vi "Spiral Search Tool.vi"(7 "Calling VI Ref":refnum<vi>) -> ()   [LabVIEW 2016]
uses:
  Hardware Configuration/Hardware Configuration Controls/Device Type.ctl
  Hardware Configuration/Hardware Configuration Controls/Device Function.ctl
  <vilib>/Utility/miscctls.llb/LVPointTypeDef.ctl
  Spiral Search Tool Type Defs/Spiral Search Tool Notifier Type.ctl
  Spiral Search Tool Type Defs/Spiral Search Tool Actions.ctl
  Device Library/Stages/Stages Controls/Stage Actions.ctl
panel:
  in  "Frames per Step":u32=1
  in  "Step Size (µm)":dbl=1.0
  in  "Camera":i32(ring) items=["Hamamatsu-Camera-Primary-0"]
  in  "Update Cameras":bool
  in  "Exit":bool
  in  "Resume Current":bool
  in  "Pause Current":bool
  in  "Start New":bool
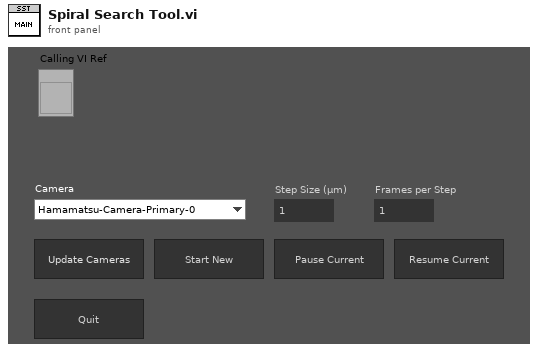
[diagram p1: front panel]
types:
  T1 = enum16{"Always On", "Always Off", "Off While Running"}
  T2 = typedef "LVPointTypeDef.ctl" = cluster{"Horizontal":i16, "Vertical":i16}
  T3 = typedef "Device Function.ctl" = enum16{"Primary", "Secondary", "Overview", "Wide Field Drift Correction", "642 nm Excitation", "560 nm Excitation", "546 nm Excitation", "488 nm Excitation", "405 nm Excitation", "Objective Drift Correction", "Objective XY", "Objective Z", "Sample XY", "Sample Coarse Z", "Sample Z", "4Pi Lower", "4Pi Upper", "Adj Cavity"}
  T4 = typedef "Device Type.ctl" = enum16{"AOTF", "Camera", "Deformable Mirror", "Laser", "Shutter", "Stage"}
  T5 = typedef "Spiral Search Tool Notifier Type.ctl" = cluster{"Actions":T6, "Camera Notifier Name":string}
  T6 = typedef "Spiral Search Tool Actions.ctl" = enum16{"Idle", "Start New", "Resume Current", "Pause Current", "Capture Image", "Move Stage", "Generate Points", "Exit"}
  T7 = typedef "Stage Actions.ctl" = enum16{"Get Position", "MVR", "MOVE", "HALT", "ONTARGET", "ERROR", "REFERENCE", "INIT", "VELOCITY", "STATUS", "EXIT", "HOME", "ZEROPOS", "NANOPOS", "ANALOG", "QUIT"}
  T8 = typedef "LVRectTypeDef.ctl" = cluster{"Left":i16, "Top":i16, "Right":i16, "Bottom":i16}
  T9 = typedef "LVBoundsTypeDef.ctl" = cluster{"Width":u32, "Height":u32}
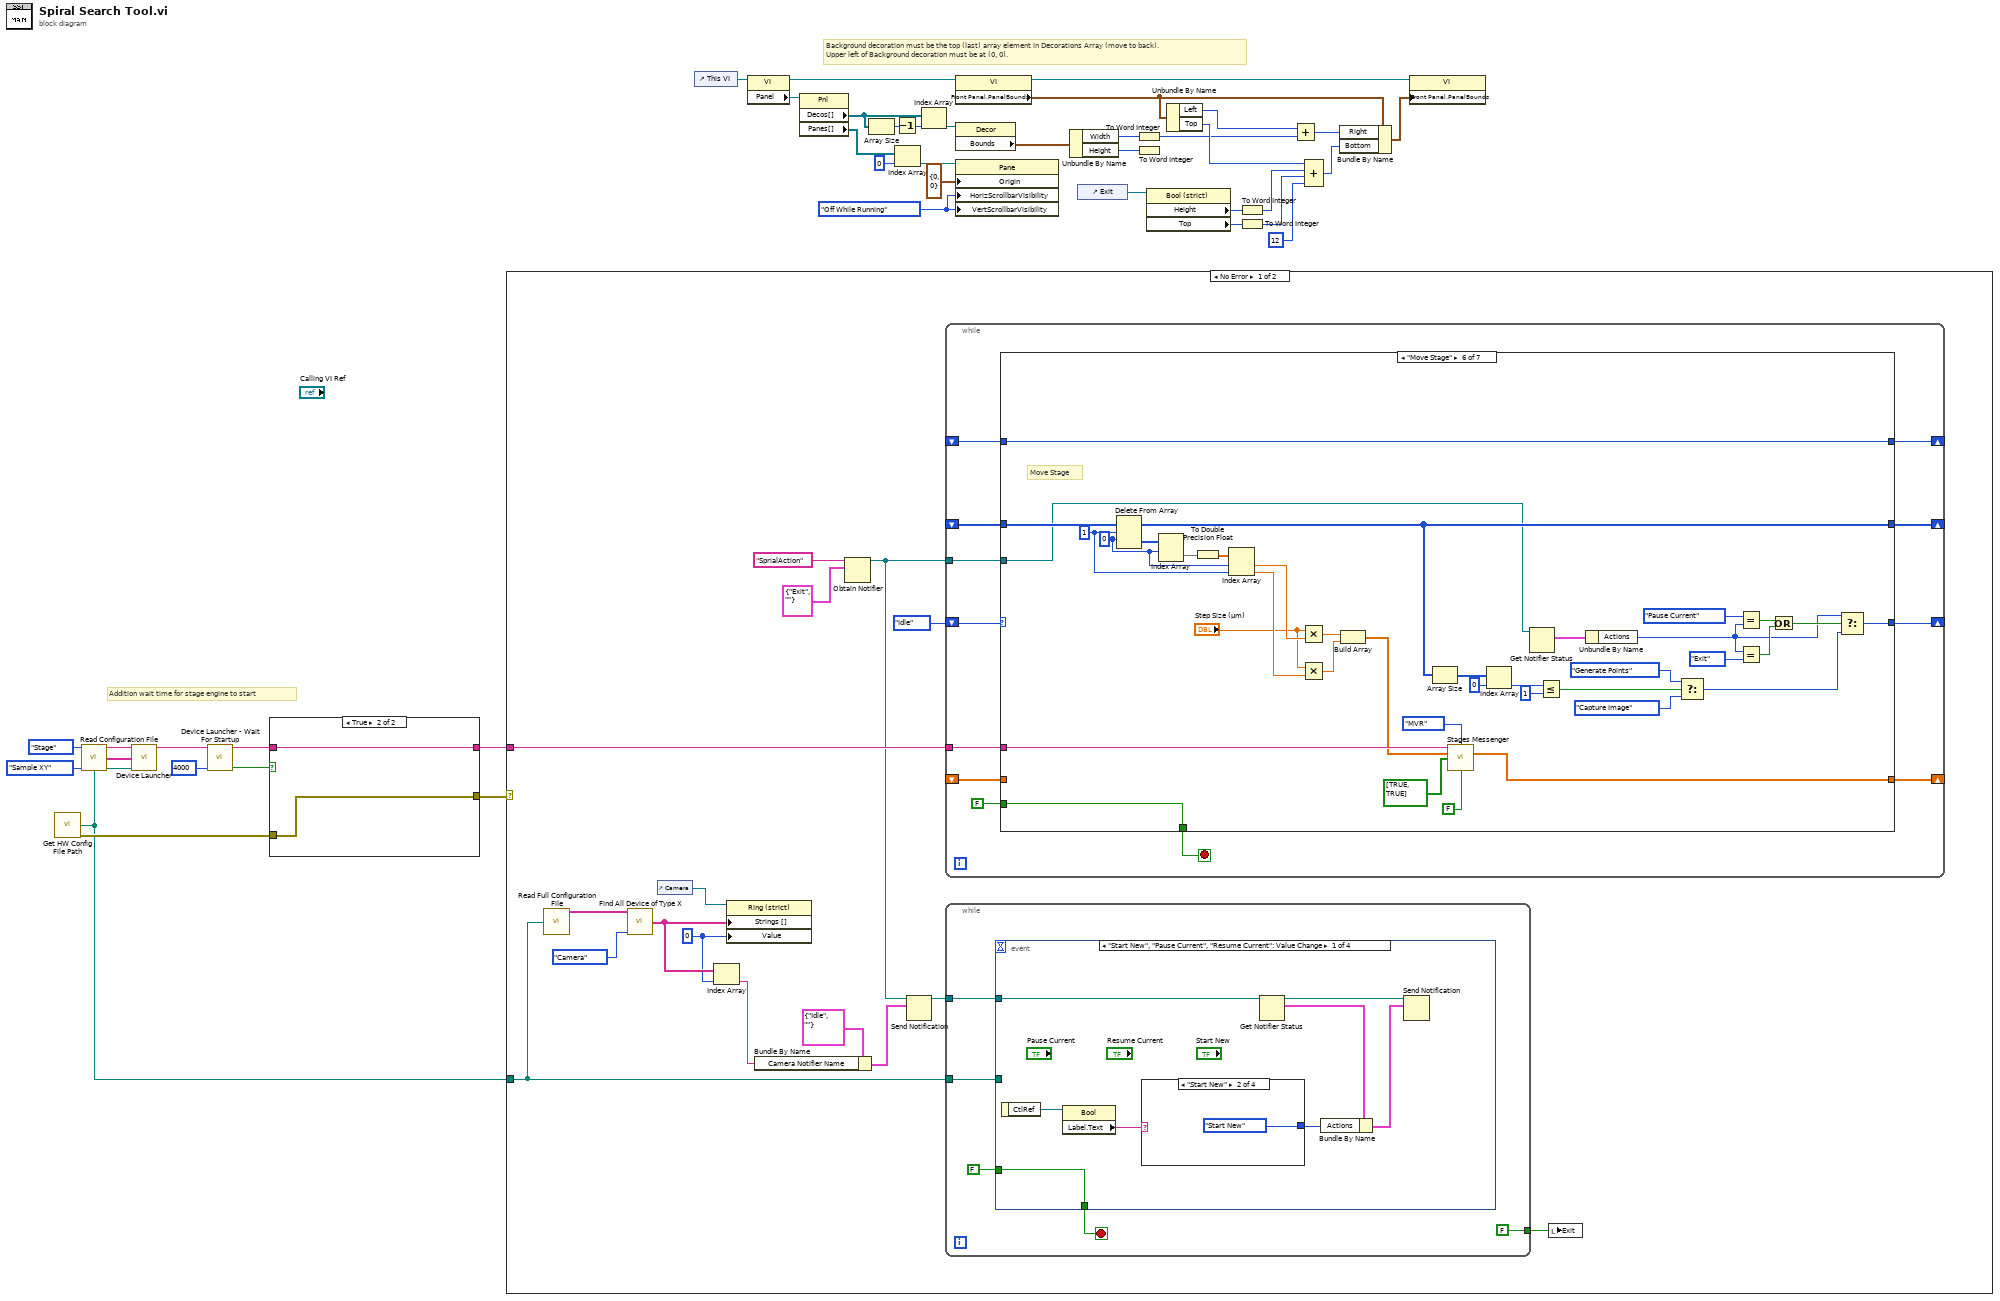
[diagram p0: block diagram]
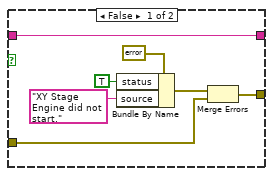
[diagram p2: hidden frame]
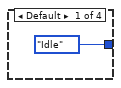
[diagram p3: hidden frame]
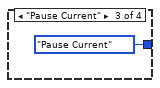
[diagram p4: hidden frame]
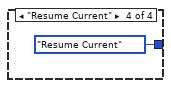
[diagram p5: hidden frame]
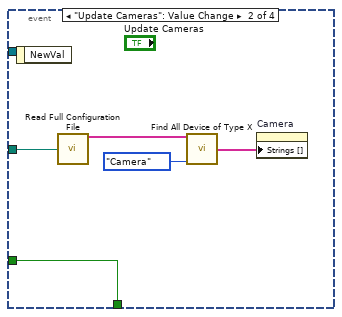
[diagram p6: hidden frame]
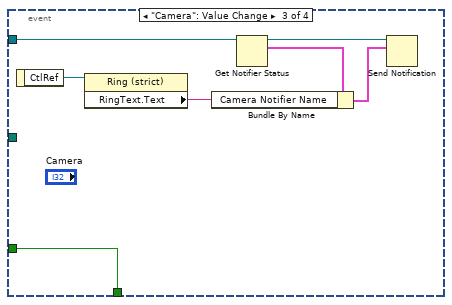
[diagram p7: hidden frame]
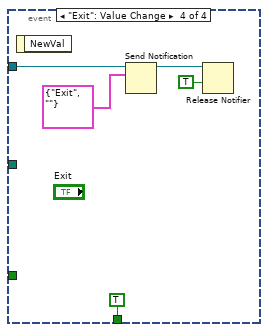
[diagram p8: hidden frame]
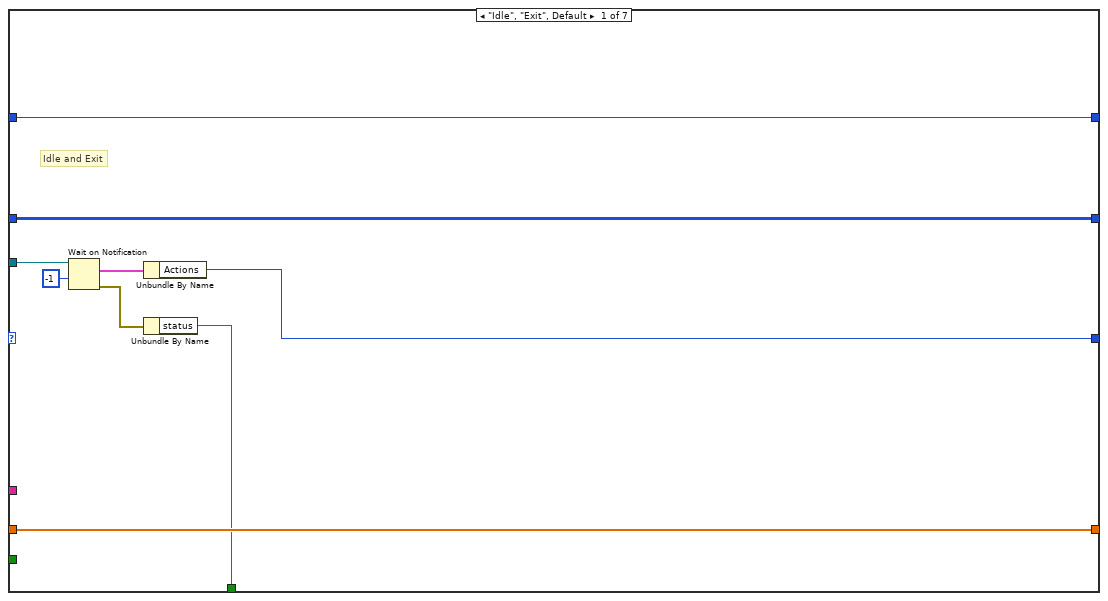
[diagram p9: hidden frame]
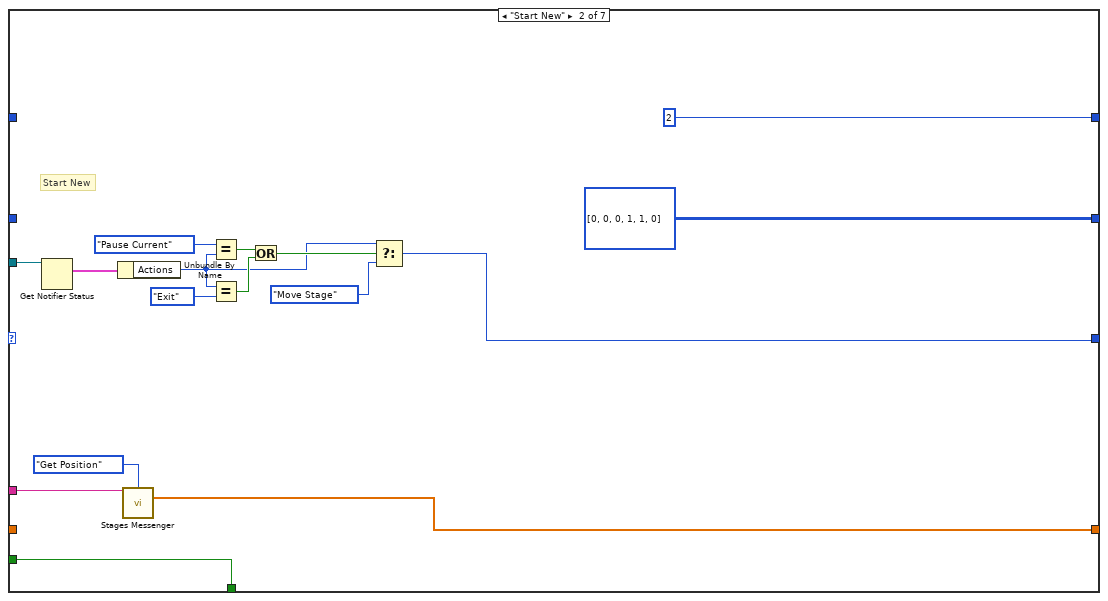
[diagram p10: hidden frame]
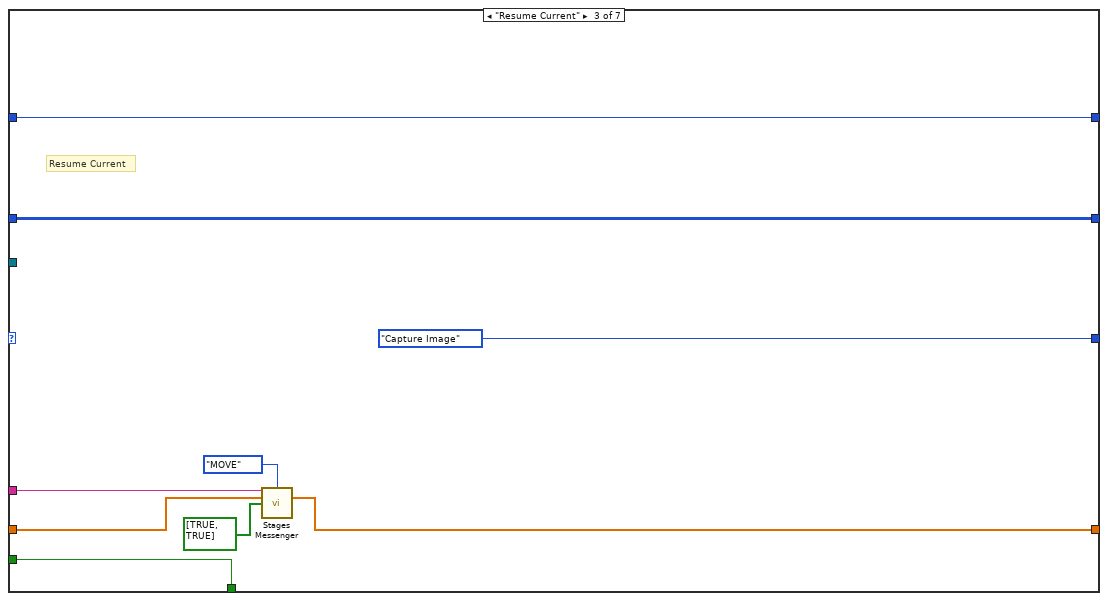
[diagram p11: hidden frame]
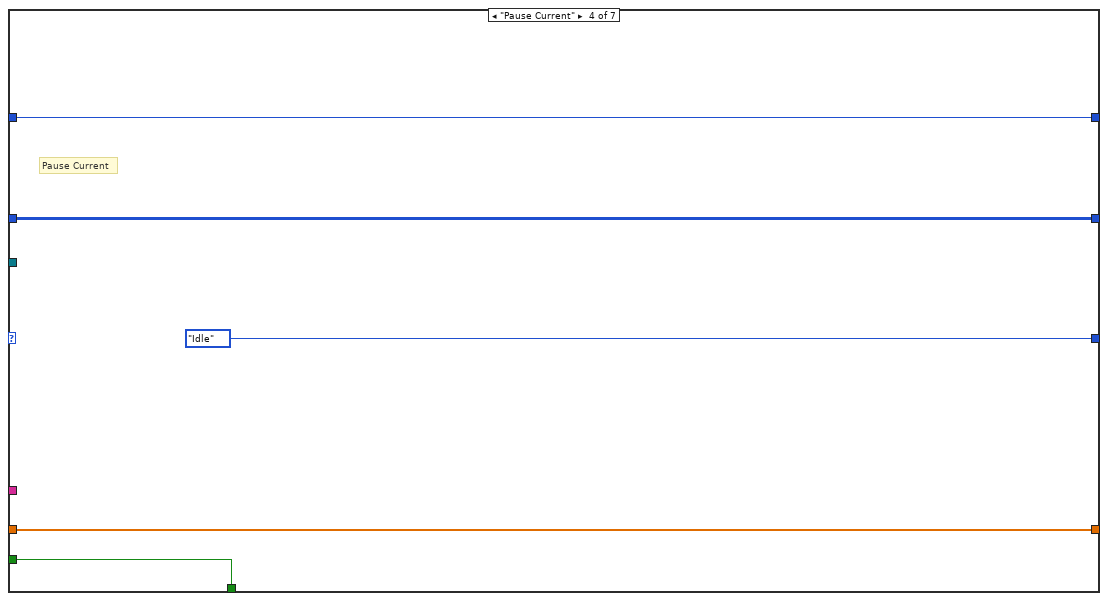
[diagram p12: hidden frame]
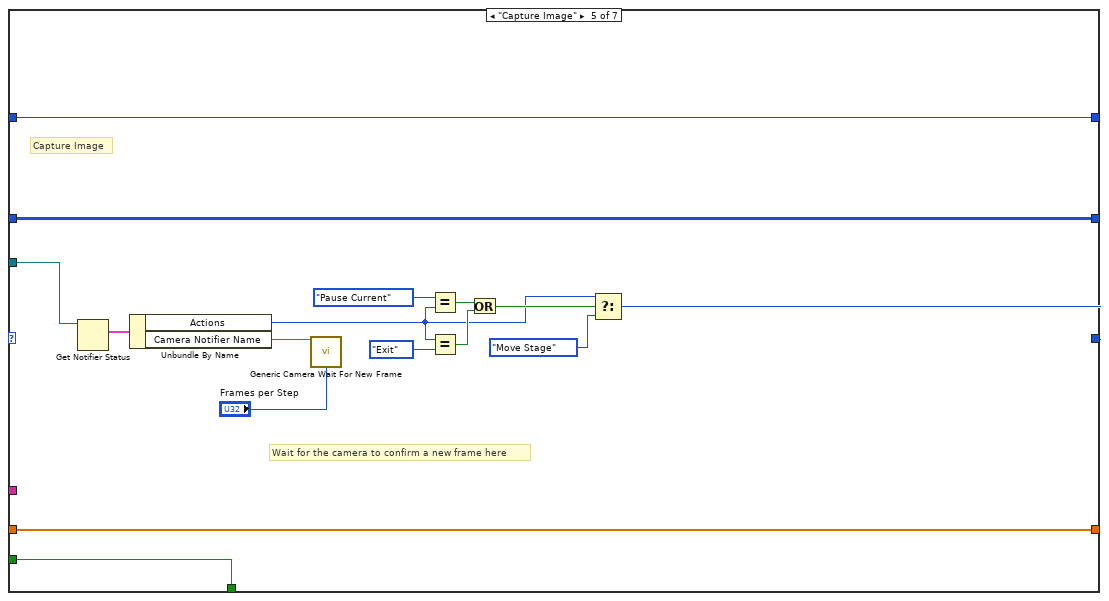
[diagram p13: hidden frame]
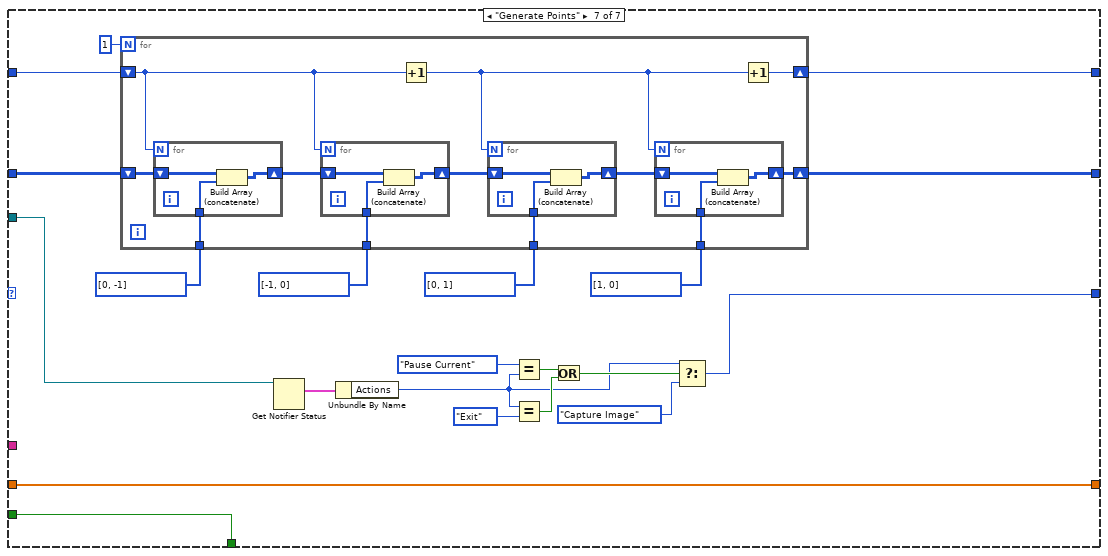
[diagram p14: hidden frame]
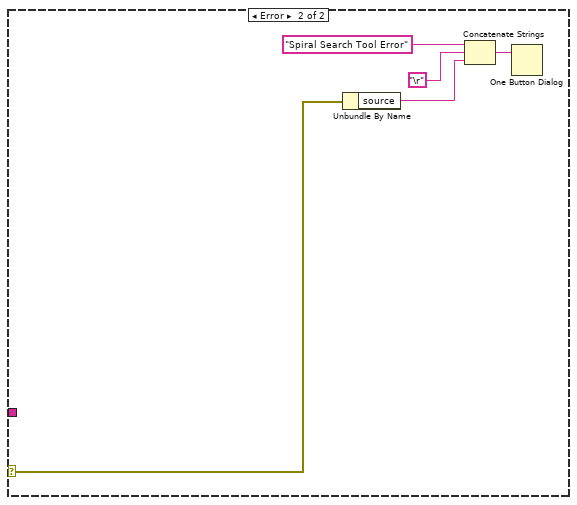
[diagram p15: hidden frame]
diagram:
  w16 = T1."Off While Running" ("Vertical Scrollbar Visibility")
  # "Addition wait time for stage engine to start"
  # "Background decoration must be the top (last) array element in Decorations Array (move to back).\nUpper left of Background decoration must be at (0, 0)."
  n1 = call "Get HW Config File Path.vi"() -> ("File Path"=w34:path, "Error"=w37:errorcluster)  [unwired: 14 in]
  n2 = call "Read Configuration File.vi"("Device Type"=Device_Type."Stage", "Device Function"=Device_Function."Sample XY", "Config File Path"=w34) -> ("Unique Notifier Name"=w42:string, "Device Ports/IDs/Channels"=w40:string[], "Device Engine Path"=w41:path)  [unwired: 9 in, 1 out]
  n3 = call "Device Launcher.vi"("Notifier Name"=w42, "Device Ports/IDs/Channels"=w40, "Device Engine Path"=w41) -> ("Notifier Name"=w4:string)  [unwired: 11 in, 1 out]
  n4 = call "Device Launcher - Wait For Startup.vi"("Notifier Name"=w4, "Wait Time (ms)"=4000) -> ("Notifier Name (Dup)"=w3:string, "Running?"=w2:bool)  [unwired: 12 in]
  n5 = case shown="True" w2 {
    tunnel: w3 -> [w49 w51]
    tunnel: [w49 w51] -> w35
    tunnel: w37 -> [w44 w50]
    tunnel: [w43 w50] -> w36
    frame False {
      n6 = Bundle By Name(cluster=errorcluster {"status"=FALSE, "code"=0, "source"=""} ("Error"), "status"=TRUE, "source"="XY Stage Engine did not start.") -> (w45:errorcluster)
      n7 = Merge Errors(w45, w44) -> (w43:errorcluster)
    }
    frame True {
    }
  }
  n8 = case shown="No Error" w36 {
    selector: w36 -> [_ w251]
    tunnel: w35 -> [w66 _]
    tunnel: w34 -> [w63 _]
    frame No Error {
      w57 = 0
      n9 = call "Read Full Configuration File.vi"("Config File Path"=w63) -> ("Unique Notifier Names"=w65:string[])  [unwired: 11 in, 3 out]
      n10 = call "Find All Device of Type X.vi"("Unique Notifier Names"=w65, "Device Type"=Device_Type."Camera") -> ("Running Devices"=w58:string[])  [unwired: 13 in]
      n11 = control-ref of="Camera"() -> (w60:refnum<vi>)
      n12 = Index Array(array=w58, index=w57) -> (element=w52:string)
      n13 = property on="Property Node" class="Ring (strict)"(reference=w60, "Strings []"=w58, "Value"=w57) -> ()  [unwired: 1 in, 2 out]
      n14 = Bundle By Name(cluster=T5 {"Actions"=enum."Idle", "Camera Notifier Name"=""} ("Spiral Search Note Type"), "Camera Notifier Name"=w52) -> (w53:T5)
      n15 = Obtain Notifier(name (unnamed)="SprialAction", notification data type=T5 {"Actions"=enum."Exit", "Camera Notifier Name"=""} ("Spiral Search Note Type")) -> (notifier out=w55:refnum<notifier>)  [unwired: 2 in, 2 out]
      n16 = Send Notification(notification=w53, notifier=w55) -> (notifier out=w54:refnum<notifier>)  [unwired: 1 in, 1 out]
      n17 = while {
        shift-right: [w109] -> _
        shift-left: _ -> [w113]
        shift-right: [w110] -> _
        shift-left: _ -> [w112]
        shift-right: [w107] -> _
        shift-left: Spiral_Search_Tool_Actions."Idle" ("Actions") -> [w111]
        tunnel: w55 -> [w108]
        shift-right: [w105] -> _
        shift-left: _ -> [w106]
        tunnel: w66 -> [w104]
        stop <- w103 stop-if-true
        n18 = case shown="\"Move Stage\"" w111 {
          tunnel: w113 -> [w120 _ w147 w152 w168 w205 w226]
          tunnel: w112 -> [w119 _ w146 w151 w167 w199 w225]
          tunnel: [w119 i8[][] [[0, 0], [0, 1], [1, 0]] w146 w151 w167 w198 w219] -> w110
          tunnel: [w120 2 w147 w152 w168 w205 w218] -> w109
          tunnel: w108 -> [w122 w136 _ _ w165 w188 w216]
          tunnel: [w115 w132 Spiral_Search_Tool_Actions."Capture Image" ("Actions") Spiral_Search_Tool_Actions."Idle" ("Actions") w155 w171 w207] -> w107
          tunnel: [w118 w131 w141 w150 w166 w186 w217] -> w105
          tunnel: w106 -> [w118 _ w143 w150 w166 _ w217]
          tunnel: w104 -> [_ w129 w144 _ _ w187 _]
          tunnel: [w116 w123 w139 w149 w153 w170 w206] -> w103
          tunnel: FALSE -> [_ w123 w139 w149 w153 w170 w206]
          frame "Idle", "Exit", Default {
            # "Idle and Exit"
            n19 = Wait on Notification(notifier=w122, timeout in ms (-1)=-1) -> (notification=w114:T5, error out=w117:errorcluster)  [unwired: 2 in, 2 out]
            n20 = Unbundle By Name(w114) -> ("Actions"=w115:T6)
            n21 = Unbundle By Name(w117) -> ("status"=w116:bool)
          }
          frame "Start New" {
            # "Start New"
            n22 = Get Notifier Status(notifier=w136) -> (current notification=w128:T5)  [unwired: 1 in, 4 out]
            n23 = Unbundle By Name(w128) -> ("Actions"=w127:T6)
            n24 = call "Stages Messenger.vi"("Stage Notifier Name"=w129, "Actions"=Stage_Actions."Get Position") -> ("Positions"=w131:dbl[])  [unwired: 10 in, 3 out]
            n25 = Equal?(x=Spiral_Search_Tool_Actions."Pause Current", y=w127) -> (x = y?=w135:bool)
            n26 = Equal?(x=w127, y=Spiral_Search_Tool_Actions."Exit") -> (x = y?=w134:bool)
            n27 = Or(x=w135, y=w134) -> (x .or. y?=w133:bool)
            n28 = Select(t=w127, s=w133, f=Spiral_Search_Tool_Actions."Move Stage") -> (s? t:f=w132:T6)
          }
          frame "Resume Current" {
            # "Resume Current"
            n29 = call "Stages Messenger.vi"("Stage Notifier Name"=w144, "Actions"=Stage_Actions."MOVE", "Setpoint"=w143, "Axis"=bool[] [TRUE, TRUE]) -> ("Positions"=w141:dbl[])  [unwired: 8 in, 3 out]
          }
          frame "Pause Current" {
            # "Pause Current"
          }
          frame "Capture Image" {
            # "Capture Image"
            # "Wait for the camera to confirm a new frame here"
            n30 = Get Notifier Status(notifier=w165) -> (current notification=w156:T5)  [unwired: 1 in, 4 out]
            n31 = Unbundle By Name(w156) -> ("Actions"=w160:T6, "Camera Notifier Name"=w154:string)
            n32 = call "Generic Camera Wait For New Frame.vi"("Camera Notifier Name"=w154, "Wait No. (1)"="Frames per Step") -> ()  [unwired: 13 in, 1 out]
            n33 = Equal?(x=Spiral_Search_Tool_Actions."Pause Current", y=w160) -> (x = y?=w163:bool)
            n34 = Equal?(x=w160, y=Spiral_Search_Tool_Actions."Exit") -> (x = y?=w162:bool)
            n35 = Or(x=w163, y=w162) -> (x .or. y?=w161:bool)
            n36 = Select(t=w160, s=w161, f=Spiral_Search_Tool_Actions."Move Stage") -> (s? t:f=w155:T6)
          }
          frame "Move Stage" {
            w195 = 0 ("index (row)")
            w194 = 1 ("length")
            # "Move Stage"
            n37 = Delete From Array(array=w199, length=w194, index (row)=w195) -> (deleted portion=w197:i8[][], array with subset deleted=w198:i8[][])  [unwired: 1 in]
            n38 = Index Array(array=w197, index (row)=w195) -> (element=w196:i8[])  [unwired: 1 in]
            n39 = To Double Precision Float(number=w196) -> (double precision float=w193:dbl[])
            n40 = Index Array(array=w193, index #1=w195, index #2=w194) -> (element #1=w192:dbl, element #2=w191:dbl)
            n41 = Multiply(x="Step Size (µm)", y=w192) -> (x*y=w190:dbl)
            n42 = Multiply(x="Step Size (µm)", y=w191) -> (x*y=w189:dbl)
            n43 = Build Array(w190, w189) -> (w182:dbl[])
            n44 = Array Size(array=w198) -> (size(s)=w204:i32[])
            n45 = call "Stages Messenger.vi"("Stage Notifier Name"=w187, "Actions"=Stage_Actions."MVR", "Setpoint"=w182, "Axis"=bool[] [TRUE, TRUE], "Exit While Busy?"=FALSE) -> ("Positions"=w186:dbl[])  [unwired: 7 in, 3 out]
            n46 = Index Array(array=w204, index=0) -> (element=w202:i32)
            n47 = Get Notifier Status(notifier=w188) -> (current notification=w174:T5)  [unwired: 1 in, 4 out]
            n48 = Less Or Equal?(x=w202, y=1) -> (x <= y?=w200:bool)
            n49 = Unbundle By Name(w174) -> ("Actions"=w173:T6)
            n50 = Select(t=Spiral_Search_Tool_Actions."Generate Points" ("f"), s=w200, f=Spiral_Search_Tool_Actions."Capture Image") -> (s? t:f=w172:T6)
            n51 = Equal?(x=Spiral_Search_Tool_Actions."Pause Current", y=w173) -> (x = y?=w181:bool)
            n52 = Equal?(x=w173, y=Spiral_Search_Tool_Actions."Exit") -> (x = y?=w180:bool)
            n53 = Or(x=w181, y=w180) -> (x .or. y?=w179:bool)
            n54 = Select(t=w173, s=w179, f=w172) -> (s? t:f=w171:T6)
          }
          frame "Generate Points" {
            n55 = for {
              N: 1 -> [_]
              shift-right: [w227] -> w218
              shift-left: w226 -> [w230]
              tunnel: i8[] [0, -1] -> [w238]
              tunnel: i8[] [-1, 0] -> [w234]
              tunnel: i8[] [0, 1] -> [w233]
              shift-right: [w228] -> w219
              shift-left: w225 -> [w232]
              tunnel: i8[] [1, 0] -> [w231]
              n56 = for {
                N: w230 -> [_]
                tunnel: w238 -> [w249]
                shift-right: [w248] -> w237
                shift-left: w232 -> [w250]
                n57 = Build Array (concatenate)(w250, w249) -> (w248:i8[][])
              }
              n58 = for {
                N: w230 -> [_]
                tunnel: w234 -> [w246]
                shift-right: [w245] -> w236
                shift-left: w237 -> [w247]
                n59 = Build Array (concatenate)(w247, w246) -> (w245:i8[][])
              }
              n60 = Increment(x=w230) -> (x+1=w229:i32)
              n61 = for {
                N: w229 -> [_]
                tunnel: w233 -> [w243]
                shift-right: [w242] -> w235
                shift-left: w236 -> [w244]
                n62 = Build Array (concatenate)(w244, w243) -> (w242:i8[][])
              }
              n63 = for {
                N: w229 -> [_]
                tunnel: w231 -> [w240]
                shift-right: [w239] -> w228
                shift-left: w235 -> [w241]
                n64 = Build Array (concatenate)(w241, w240) -> (w239:i8[][])
              }
              n65 = Increment(x=w229) -> (x+1=w227:i32)
            }
            n66 = Get Notifier Status(notifier=w216) -> (current notification=w215:T5)  [unwired: 1 in, 4 out]
            n67 = Unbundle By Name(w215) -> ("Actions"=w208:T6)
            n68 = Equal?(x=Spiral_Search_Tool_Actions."Pause Current", y=w208) -> (x = y?=w214:bool)
            n69 = Equal?(x=w208, y=Spiral_Search_Tool_Actions."Exit") -> (x = y?=w213:bool)
            n70 = Or(x=w214, y=w213) -> (x .or. y?=w212:bool)
            n71 = Select(t=w208, s=w212, f=Spiral_Search_Tool_Actions."Capture Image") -> (s? t:f=w207:T6)
          }
        }
      }
      n72 = while {
        tunnel: w54 -> [w72]
        tunnel: w63 -> [w69]
        tunnel: [FALSE] -> w59
        stop <- w70 stop-if-true
        n73 = event shown="[0] \"Start New\", \"Pause Current\", \"Resume Current\": Value Change" {
          selector: _ -> [_ _ _ _]
          dyn-events: _ -> [_ _ _ _]
          timeout: _ -> [_ _ _ _]
          tunnel: w72 -> [w77 _ w94 w101]
          tunnel: FALSE -> [w80 w89 w96 _]
          tunnel: [w80 w89 w96 TRUE] -> w70
          tunnel: w69 -> [_ w88 _ _]
          event "Start New", "Pause Current", "Resume Current": Value Change {
            n74 = event-data() -> ("CtlRef"=w79:refnum<vi>)  [unwired: 1 in]
            n75 = property class="Bool"(reference=w79) -> ("Label.Text"=w78:string)  [unwired: 1 in, 2 out]
            n76 = case shown="\"Start New\"" w78 {
              tunnel: [Spiral_Search_Tool_Actions."Idle" ("Actions") Spiral_Search_Tool_Actions."Start New" ("Actions") Spiral_Search_Tool_Actions."Pause Current" ("Actions") Spiral_Search_Tool_Actions."Resume Current" ("Actions")] -> w74
              frame Default {
              }
              frame "Start New" {
              }
              frame "Pause Current" {
              }
              frame "Resume Current" {
              }
            }
            n77 = Get Notifier Status(notifier=w77) -> (notifier out=w76:refnum<notifier>, current notification=w75:T5)  [unwired: 1 in, 3 out]
            n78 = Bundle By Name(cluster=w75, "Actions"=w74) -> (w73:T5)
            n79 = Send Notification(notification=w73, notifier=w76) -> ()  [unwired: 1 in, 2 out]
          }
          event "Update Cameras": Value Change {
            n80 = event-data() -> ()  [unwired: 1 in, 1 out]
            n81 = call "Read Full Configuration File.vi"("Config File Path"=w88) -> ("Unique Notifier Names"=w87:string[])  [unwired: 11 in, 3 out]
            n82 = call "Find All Device of Type X.vi"("Unique Notifier Names"=w87, "Device Type"=Device_Type."Camera") -> ("Running Devices"=w85:string[])  [unwired: 13 in]
            n83 = property on="Camera" class="Ring (strict)"("Strings []"=w85) -> ()  [unwired: 2 in, 2 out]
          }
          event "Camera": Value Change {
            n84 = event-data() -> ("CtlRef"=w95:refnum<vi>)  [unwired: 1 in]
            n85 = property class="Ring (strict)"(reference=w95) -> ("RingText.Text"=w90:string)  [unwired: 1 in, 2 out]
            n86 = Get Notifier Status(notifier=w94) -> (notifier out=w93:refnum<notifier>, current notification=w92:T5)  [unwired: 1 in, 3 out]
            n87 = Bundle By Name(cluster=w92, "Camera Notifier Name"=w90) -> (w91:T5)
            n88 = Send Notification(notification=w91, notifier=w93) -> ()  [unwired: 1 in, 2 out]
          }
          event "Exit": Value Change {
            n89 = event-data() -> ()  [unwired: 1 in, 1 out]
            n90 = Send Notification(notification=T5 {"Actions"=enum."Exit", "Camera Notifier Name"=""}, notifier=w101) -> (notifier out=w99:refnum<notifier>)  [unwired: 1 in, 1 out]
            n91 = Release Notifier(notifier=w99, force destroy? (F)=TRUE) -> ()  [unwired: 1 in, 3 out]
          }
        }
      }
      n92 = local write "Exit"(w59) -> ()
    }
    frame Error {
      n93 = Unbundle By Name(w251) -> ("source"=w253:string)
      n94 = Concatenate Strings("Spiral Search Tool Error", "\r", w253) -> (w252:string)
      n95 = One Button Dialog(message=w252) -> ()  [unwired: 1 in, 1 out]
    }
  }
  n96 = control-ref of="This VI"() -> (w9:refnum<vi>)
  n97 = property class="VI"(reference=w9) -> (reference out=w17:refnum<vi>, "Panel"=w10:refnum<vi>)  [unwired: 1 in, 1 out]
  n98 = property class="Pnl"(reference=w10) -> ("Decos[]"=w8:refnum<vi>[], "Panes[]"=w13:refnum<vi>[])  [unwired: 1 in, 2 out]
  n99 = Array Size(array=w8) -> (size(s)=w6:i32)
  n100 = Decrement(x=w6) -> (x-1=w7:i32)
  n101 = Index Array(array=w13, index=0) -> (element=w12:refnum<vi>)
  n102 = Index Array(array=w8, index=w7) -> (element=w15:refnum<vi>)
  n103 = property class="VI"(reference=w17) -> (reference out=w19:refnum<vi>, "Front Panel.PanelBounds"=w20:T8)  [unwired: 1 in, 1 out]
  n104 = property class="Decor"(reference=w15) -> ("Bounds"=w18:T9)  [unwired: 1 in, 2 out]
  n105 = property class="Pane"(reference=w12, "Origin"=T2 {"Horizontal"=0, "Vertical"=0}, "HorizScrollbarVisibility"=w16, "VertScrollbarVisibility"=w16) -> ()  [unwired: 1 in, 2 out]
  n106 = Unbundle By Name(w18) -> ("Width"=w23:u32, "Height"=w26:u32)
  n107 = control-ref of="Exit"() -> (w5:refnum<vi>)
  n108 = To Word Integer(number=w23) -> (16bit integer=w25:i16)
  n109 = To Word Integer(number=w26) -> ()  [unwired: 1 out]
  n110 = property class="Bool (strict)"(reference=w5) -> ("Height"=w28:u32, "Top"=w29:i32)  [unwired: 1 in, 2 out]
  n111 = Unbundle By Name(w20) -> ("Left"=w22:i16, "Top"=w33:i16)
  n112 = To Word Integer(number=w28) -> (16bit integer=w31:i16)
  n113 = To Word Integer(number=w29) -> (16bit integer=w32:i16)
  n114 = Add(x=w22, y=w25) -> (x+y=w24:i16)
  n115 = Compound Arithmetic op=ADD(w33, w31, w32, i16 12 ("y")) -> (w27:i16)
  n116 = Bundle By Name(cluster=w20, "Right"=w24, "Bottom"=w27) -> (w21:T8)
  n117 = property class="VI"(reference=w19, "Front Panel.PanelBounds"=w21) -> ()  [unwired: 1 in, 2 out]
